vi "DMSU.messages.vi"(1 "message":string, 2 "errorMessage":errorcluster, 4 "Action":T1(ring), 5 "error in (no error)":errorcluster) -> (15 "messages":string[](array[string]), 19 "error out":errorcluster)   [LabVIEW 2014, in "DMSUtils.lvlib"]
doc: "primivite handler for messages"
uses:
  DMSUtils.lvlib
  <vilib>/Utility/error.llb/DialogType.ctl
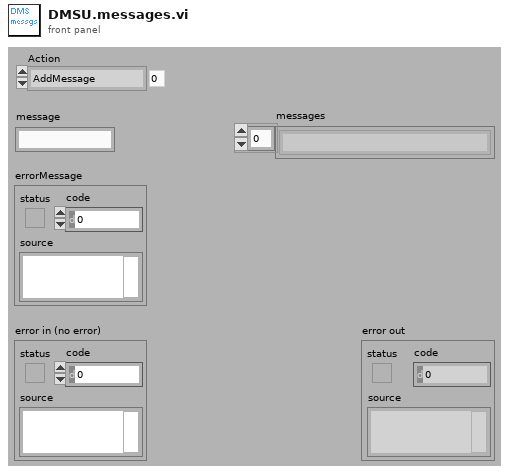
[diagram p1: front panel]
types:
  T1 = enum16{"AddMessage", "AddErrorMessage", "GetMessages"}
  T2 = typedef "DialogType.ctl" = u16
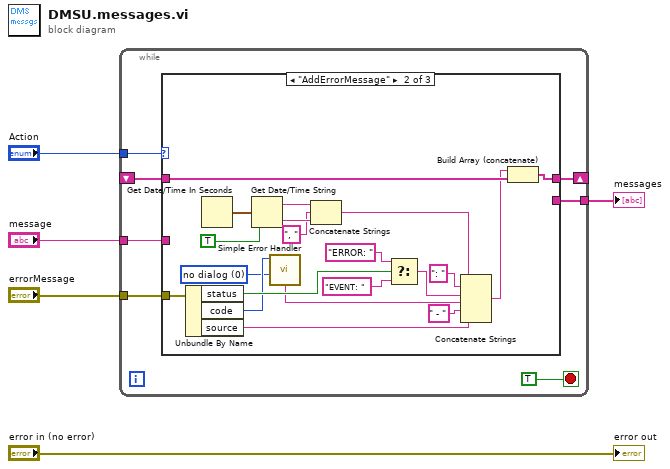
[diagram p0: block diagram]
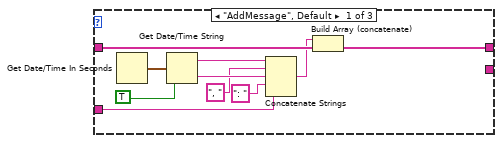
[diagram p2: hidden frame]
diagram:
  n1 = while {
    tunnel: "Action" -> [w11]
    shift-right: [w8] -> _
    shift-left: _ -> [w10]
    tunnel: "message" -> [w9]
    tunnel: [w7] -> w3
    tunnel: "errorMessage" -> [w6]
    stop <- TRUE stop-if-true
    n2 = case shown="\"AddErrorMessage\"" w11 {
      tunnel: w10 -> [w22 w42 w43]
      tunnel: w9 -> [w16 _ _]
      tunnel: [w21 w41 _] -> w8
      tunnel: [_ _ w43] -> w7
      tunnel: w6 -> [_ w40 _]
      frame "AddMessage", Default {
        n3 = Get Date/Time In Seconds() -> (seconds since 1Jan1904=w20:timestamp)
        n4 = Get Date/Time String(seconds (now)=w20, want seconds? (F)=TRUE) -> (date string=w19:string, time string=w18:string)  [unwired: 1 in]
        n5 = Concatenate Strings(w19, ", " ("string"), w18, ": " ("string"), w16) -> (w14:string)
        n6 = Build Array (concatenate)(w14, w22) -> (w21:string[])
      }
      frame "AddErrorMessage" {
        w31 = T2 0 items=["no dialog", "OK message", "continue or stop message", "OK message + warnings", "continue/stop + warnings"] ("type of dialog (OK msg:1)")
        n7 = Unbundle By Name(w40) -> ("status"=w38:bool, "code"=w33:i32, "source"=w34:string)
        n8 = Get Date/Time In Seconds() -> (seconds since 1Jan1904=w30:timestamp)
        n9 = Get Date/Time String(seconds (now)=w30, want seconds? (F)=TRUE) -> (date string=w28:string, time string=w27:string)  [unwired: 1 in]
        n10 = call <vilib>:"Simple Error Handler.vi"("error code (no error:0)"=w33, "type of dialog (OK msg:1)"=w31) -> ("message"=w32:string)  [unwired: 3 in, 4 out]
        n11 = Concatenate Strings(w28, ", " ("string"), w27) -> (w25:string)
        n12 = Select(t="ERROR: ", s=w38, f="EVENT: ") -> (s? t:f=w36:string)
        n13 = Concatenate Strings(w25, ": " ("string"), w36, w32, " - " ("string"), w34) -> (w23:string)
        n14 = Build Array (concatenate)(w23, w42) -> (w41:string[])
      }
      frame "GetMessages" {
      }
    }
  }
  "messages" <- w3
  "error out" <- "error in (no error)"
